vi "Close VI Front Panel.vi"(4 "Error In":errorcluster, 7 "When":enum16{"Always", "Not Development"}(ring)) -> (0 "Error Out":errorcluster)   [LabVIEW 2014, in "User Interface.lvlib"]
uses:
  User Interface.lvlib
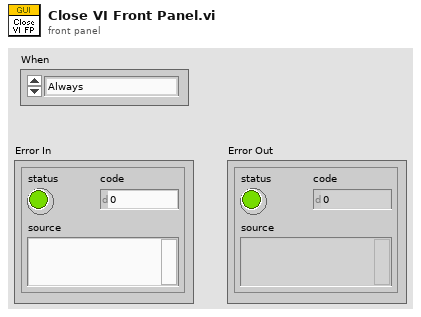
[diagram p1: front panel]
types:
  T1 = enum32{"invalid app kind", "Development System", "Run Time System", "Student Edition", "Embedded LabVIEW", "Evaluation", "Custom"}
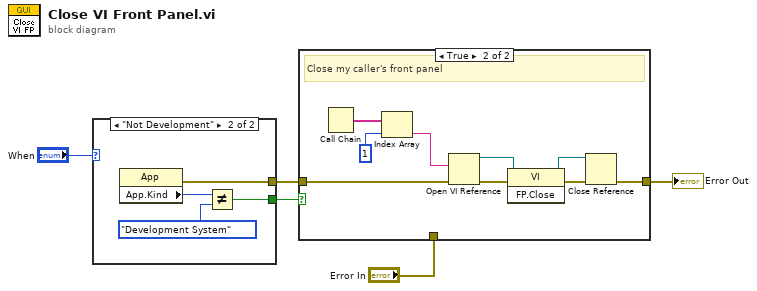
[diagram p0: block diagram]
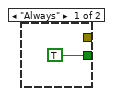
[diagram p3: hidden frame]
diagram:
  n1 = case shown="\"Not Development\"" "When" {
    tunnel: [TRUE w8] -> w3
    tunnel: [_ w7] -> w4
    frame "Always" {
    }
    frame "Not Development" {
      n2 = property class="App"() -> (error out=w7:errorcluster, "App.Kind"=w10:T1)  [unwired: 2 in, 1 out]
      n3 = Not Equal?(x=w10, y=T1."Development System") -> (x != y?=w8:bool)
    }
  }
  n4 = case shown="True" w3 {
    tunnel: w4 -> [_ w17]
    tunnel: [w11 w12] -> w2
    tunnel: "Error In" -> [w11 _]
    frame False {
      # "Do Nothing"
    }
    frame True {
      # "Close my caller's front panel"
      n5 = Call Chain() -> (call chain=w20:string[])
      n6 = Index Array(array=w20, index=1) -> (element=w18:string)
      n7 = Open VI Reference(vi path=w18, error in (no error)=w17) -> (vi reference=w15:refnum<vi>, error out=w16:errorcluster)  [unwired: 4 in]
      n8 = invoke class="VI" method="FP.Close"(reference=w15, error in=w16) -> (reference out=w13:refnum<vi>, error out=w14:errorcluster)  [unwired: 1 in, 1 out]
      n9 = Close Reference(reference=w13, error in (no error)=w14) -> (error out=w12:errorcluster)
    }
  }
  "Error Out" <- w2
